vi "PmGetCameras.vi"(8 "error in (no error)":errorcluster, 11 "Library":refnum<k24>) -> (0 "error out":errorcluster, 2 "Cameras":variant[](array[variant]), 3 "Library 2":refnum<k24>, 4 "SN":string[](array[string]), 6 "Model":string)   [LabVIEW 2022 SP3, in "Photometrics Camera.lvlib"]
uses:
  Photometrics Camera.lvlib
  C:/FlashGordon/Development/dll/PVCamNET.dll
  dll/PVCamNET.dll
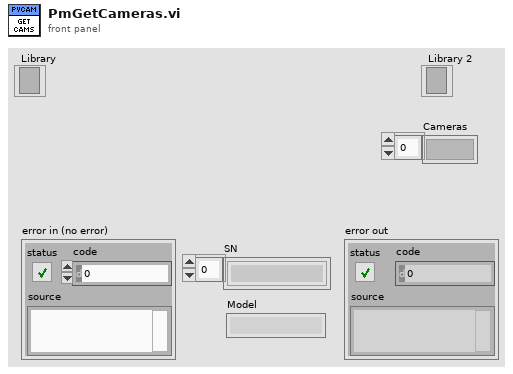
[diagram p1: front panel]
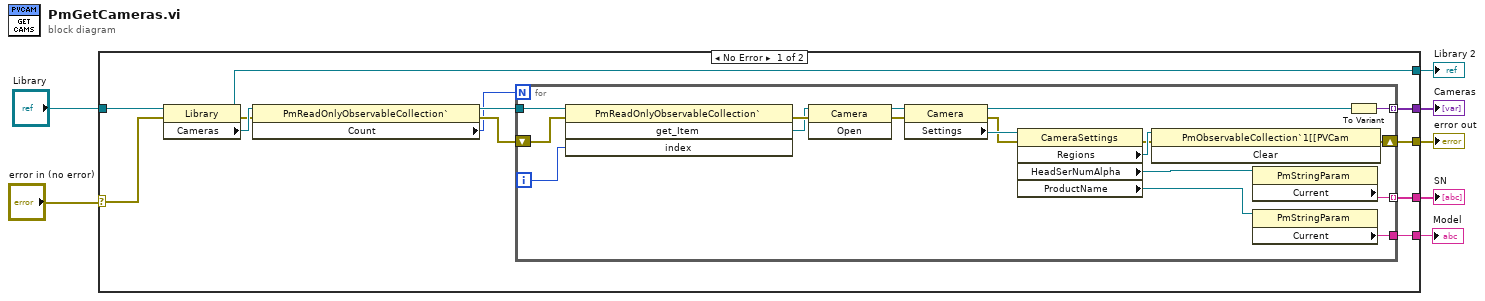
[diagram p0: block diagram]
diagram:
  n1 = case shown="No Error" "error in (no error)" {
    selector: "error in (no error)" -> [w11 w39]
    tunnel: [w19 _] -> w7
    tunnel: [w18 w39] -> w6
    tunnel: "Library" -> [w12 w38]
    tunnel: [w10 _] -> w3
    tunnel: [w9 _] -> w1
    tunnel: [w8 w38] -> w2
    frame No Error {
      n2 = property class="Library"(reference=w12, error in=w11) -> (reference out=w8:refnum<k24>, error out=w13:errorcluster, "Cameras"=w14:refnum<k24>)
      n3 = property class="PmReadOnlyObservableCollection`"(reference=w14, error in=w13) -> (reference out=w17:refnum<k24>, error out=w16:errorcluster, "Count"=w15:i32)
      n4 = for {
        N: w15 -> [_]
        tunnel: w17 -> [w37]
        tunnel: [w21] -> w19 mode=indexing
        shift-right: [w23] -> w18
        shift-left: w16 -> [w35]
        tunnel: [w31] -> w10 mode=indexing
        tunnel: [w29] -> w9
        i -> [w36]
        n5 = invoke class="PmReadOnlyObservableCollection`" method="get_Item"(reference=w37, error in=w35, "index"=w36) -> (error out=w34:errorcluster, "get_Item"=w26:refnum<k24>)  [unwired: 1 in, 2 out]
        n6 = invoke class="Camera" method="Open"(reference=w26, error in=w34) -> (reference out=w27:refnum<k24>, error out=w33:errorcluster)  [unwired: 1 in, 1 out]
        n7 = property class="Camera"(reference=w27, error in=w33) -> (reference out=w20:refnum<k24>, error out=w28:errorcluster, "Settings"=w32:refnum<k24>)
        n8 = property class="CameraSettings"(reference=w32, error in=w28) -> (error out=w22:errorcluster, "Regions"=w24:refnum<k24>, "HeadSerNumAlpha"=w25:refnum<k24>, "ProductName"=w30:refnum<k24>)  [unwired: 1 out]
        n9 = invoke class="PmObservableCollection`1[[PVCam" method="Clear"(reference=w24, error in=w22) -> (error out=w23:errorcluster)  [unwired: 1 in, 2 out]
        n10 = property class="PmStringParam"(reference=w25) -> ("Current"=w31:string)  [unwired: 1 in, 2 out]
        n11 = property class="PmStringParam"(reference=w30) -> ("Current"=w29:string)  [unwired: 1 in, 2 out]
        n12 = To Variant(anything=w20) -> (Variant=w21:variant)
      }
    }
    frame Error {
    }
  }
  "Cameras" <- w7
  "error out" <- w6
  "SN" <- w3
  "Library 2" <- w2
  "Model" <- w1
